vi "FCS_Automatic_Filename_sub.vi"(1 "bin / ns":i32, 2 "FCS save directory":path, 3 "file path":path) -> (0 "FCS output path":path)   [LabVIEW 2009]
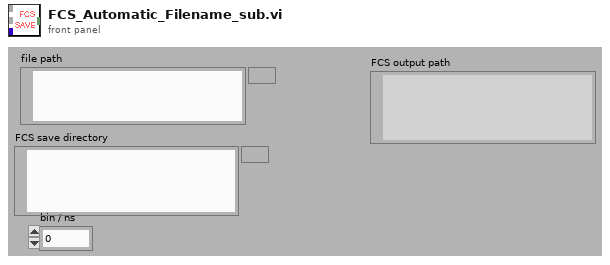
[diagram p1: front panel]
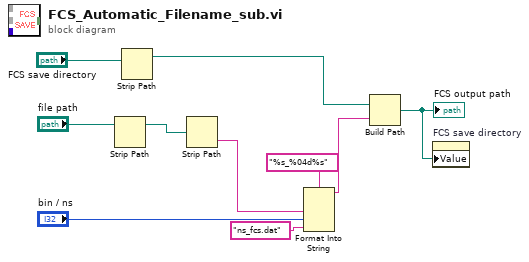
[diagram p0: block diagram]
diagram:
  n1 = Strip Path(path="file path") -> (stripped path=w9:path)  [unwired: 1 out]
  n2 = Strip Path(path="FCS save directory") -> (stripped path=w4:path)  [unwired: 1 out]
  n3 = Strip Path(path=w9) -> (name=w7:string)  [unwired: 1 out]
  n4 = Format Into String(format string="%s_%04d%s", w7, "bin / ns", "ns_fcs.dat" ("input 2")) -> (resulting string=w3:string)  [unwired: 2 in, 1 out]
  n5 = Build Path(base path=w4, name or relative path=w3) -> (appended path=w2:path)
  "FCS output path" <- w2
  n6 = property on="FCS save directory" class="Path"("Value"=w2) -> ()  [unwired: 2 in, 2 out]
